vi "Close_port.vi"(8 "error in (no error)":errorcluster, 11 "LifterTCP in":refnum<class "LifterTCP.lvclass">) -> (0 "error out":errorcluster)   [LabVIEW 2019, in "LifterTCP.lvclass"]
uses:
  LifterTCP.lvclass
  LifterTCP.lvclass/LifterTCP.ctl
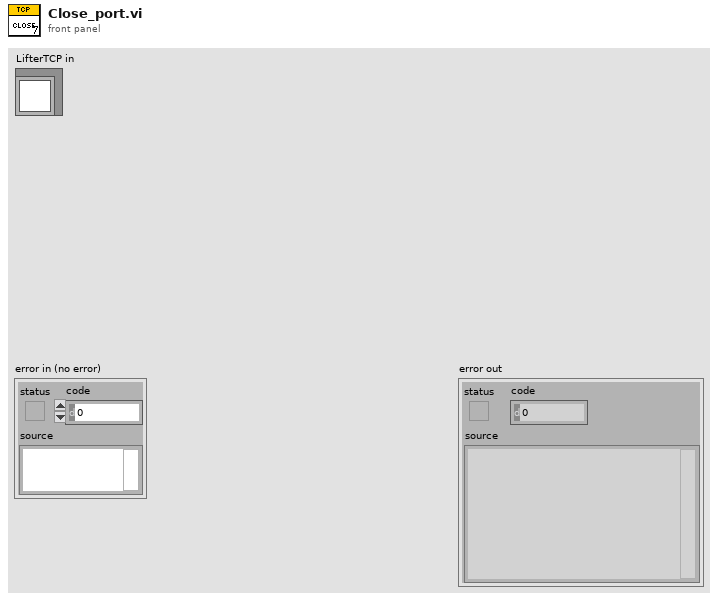
[diagram p1: front panel]
types:
  T1 = typedef "Semaphore RefNum" = refnum<k1>
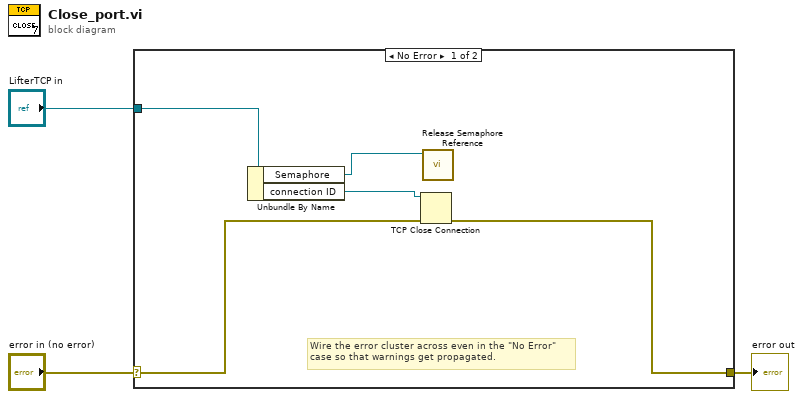
[diagram p0: block diagram]
diagram:
  n1 = case shown="No Error" "error in (no error)" {
    selector: "error in (no error)" -> [w6 w9]
    tunnel: [w4 w9] -> w2
    tunnel: "LifterTCP in" -> [w8 _]
    frame No Error {
      # "Wire the error cluster across even in the \"No Error\"\ncase so that warnings get propagated."
      n2 = Unbundle By Name(w8) -> ("Semaphore"=w5:T1, "connection ID"=w7:refnum<k5>)
      n3 = TCP Close Connection(connection ID=w7, error in (no error)=w6) -> (error out=w4:errorcluster)  [unwired: 1 in, 1 out]
      n4 = call <vilib>:"Release Semaphore Reference.vi"("semaphore"=w5) -> ()  [unwired: 9 in, 2 out]
    }
    frame Error {
    }
  }
  "error out" <- w2
